vi "apply_cal.vi"(9 "High/low index":i32, 10 "Calibration":T1 {"r bias" format="%_3p"; "Ks" format="%#_3p"}, 11 "V":dbl[](array[numeric])) -> (3 "r":dbl[](array[numeric]))   [LabVIEW 2014]
uses:
  calibration.ctl
panel:
  # "The calibration is in a somewhat inconsistent state because of partially implemented support for the YZ carriers.  See comment in vector-to-calibration."
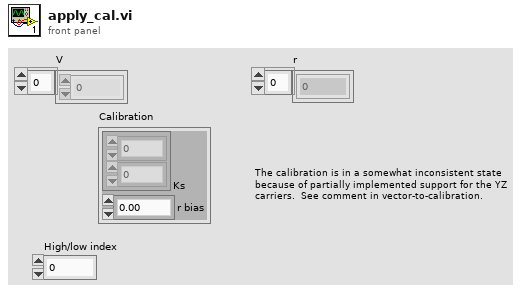
[diagram p1: front panel]
types:
  T1 = typedef "calibration.ctl" = cluster{"Ks":dbl[], "r bias":dbl}
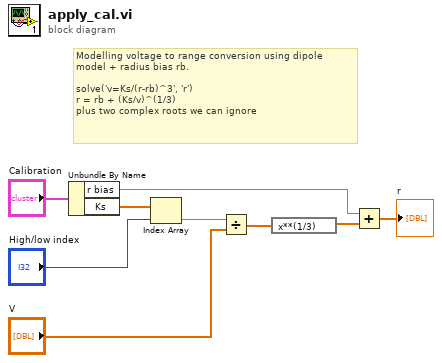
[diagram p0: block diagram]
diagram:
  # "Modelling voltage to range conversion using dipole model + radius bias rb.\n \nsolve('v=Ks/(r-rb)^3', 'r')\nr = rb + (Ks/v)^(1/3)\nplus two complex roots we can ignore"
  n1 = Unbundle By Name("Calibration") -> ("r bias"=w5:dbl, "Ks"=w3:dbl[])
  n2 = Index Array(array=w3, index="High/low index") -> (element=w2:dbl)
  n3 = Divide(x=w2, y="V") -> (x/y=w7:dbl[])
  n4 = expression code="x**(1/3)"(w7) -> (w6:dbl[])
  n5 = Add(x=w5, y=w6) -> (x+y=→"r":dbl[])
